vi "LinearPlntInvFF_New.vi"(5 "States":i32, 6 "dT_Seconds":dbl=0.02, 7 "Inputs":i32, 10 "B":T1, 11 "A":T1) -> (0 "Error":bool, 3 "Linear Plnt Inversion FF":T2)   [LabVIEW 2019, in "Trajectory_Library.lvlib"]
doc: "Creates a new LINEAR PLANT INVERSION FEEDFORWARD data cluster with the specified values. \n\n\nInputs: \n - XXX -- XXX.\n\nOutputs:\n - XXX -- XXX."
uses:
  Trajectory_Library.lvlib
  LINEAR_PLANT_INV_FF.ctl
  <vilib>/Analysis/Matrix/Datatypes/RealMatrix.ctl
  <vilib>/Analysis/Matrix/Numeric/Multiply/Multiply.vi
  <vilib>/Analysis/Matrix/Numeric/Multiply/Multiply - RM,R.vi
  Matrix_AssignBlock.vi
  Matrix_Exp.vi
  Matrix_ExtractFrom.vi
  <vilib>/Analysis/Matrix/NI_Matrix.lvlib
panel:
  # "<States,1>"
  # "<Inputs,1>"
  # "<States,Inputs>"
  # "<States,States>"
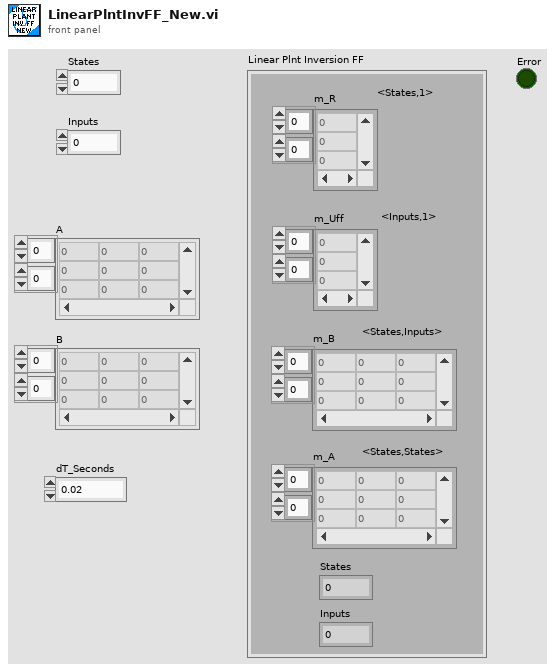
[diagram p1: front panel]
types:
  T1 = typedef "NI_Matrix.lvlib/RealMatrix.ctl" = dbl[][]
  T2 = typedef "Trajectory_Library.lvlib/LINEAR_PLANT_INV_FF.ctl" = cluster{"m_R":T1, "m_Uff":T1, "m_B":T1, "m_A":T1, "States":i32, "Inputs":i32}
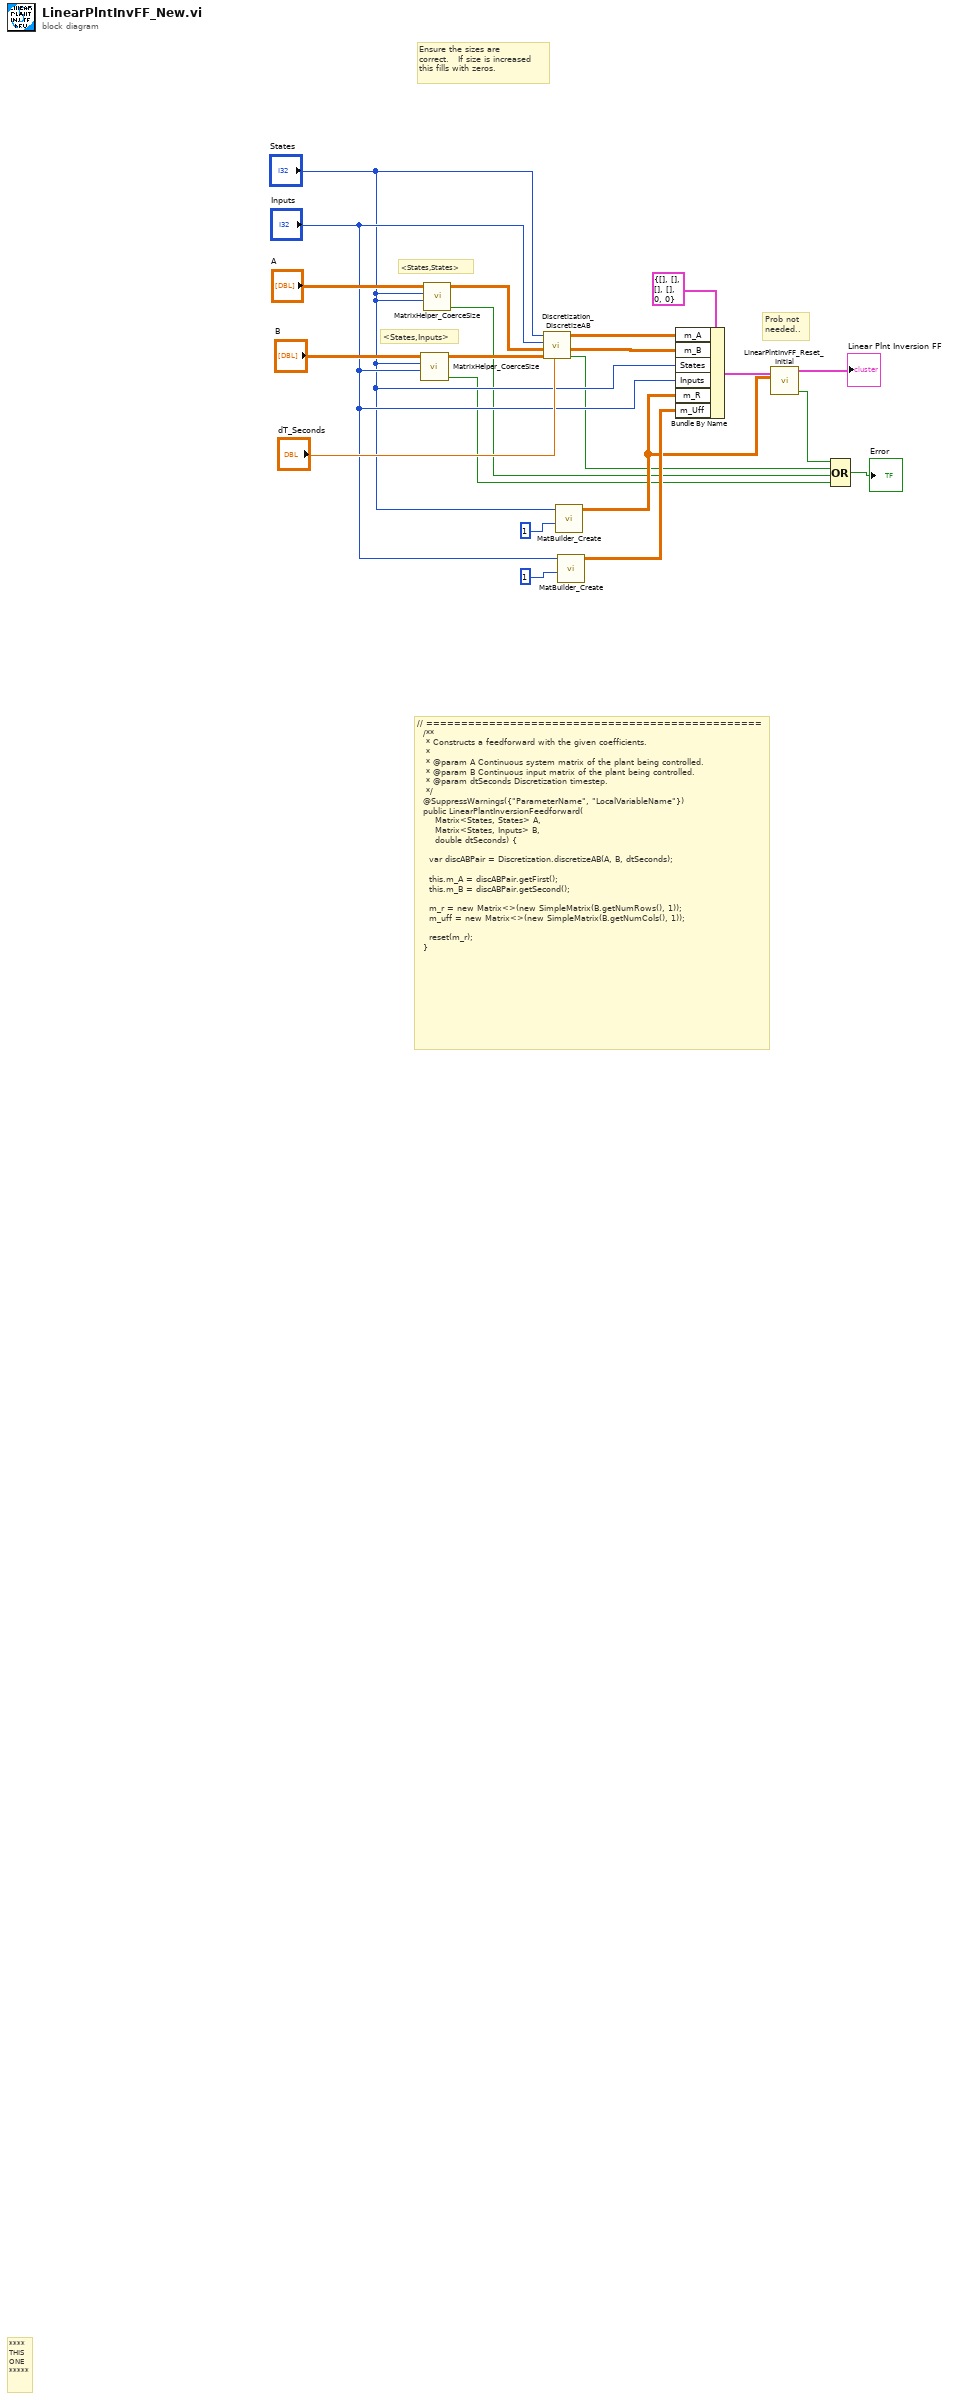
[diagram p0: block diagram]
diagram:
  # "Prob not \nneeded.."
  # "// ================================================\n  /**\n   * Constructs a feedforward with the given coefficients.\n   *\n   * @param A Continuous system matrix of the plant being controlled.\n   * @param B Continuous input matrix of the plant being controlled.\n   * @param dtSeconds Discretization timestep.\n   */\n  @SuppressWarnings({\"ParameterName\", \"LocalVariableName\"})\n  public LinearPlantInversionFeedforward(\n      Matrix<States, States> A, \n      Matrix<States, Inputs> B, \n      double dtSeconds) {\n\n    var discABPair = Discretization.discretizeAB(A, B, dtSeconds);\n \n    this.m_A = discABPair.getFirst();\n    this.m_B = discABPair.getSecond();\n\n    m_r = new Matrix<>(new SimpleMatrix(B.getNumRows(), 1));\n    m_uff = new Matrix<>(new SimpleMatrix(B.getNumCols(), 1));\n\n    reset(m_r);\n  }"
  # "<States,Inputs>"
  # "<States,States>"
  # "Ensure the sizes are\ncorrect.   If size is increased \nthis fills with zeros."
  # "****\nTHIS\nONE\n*****"
  n1 = call "MatrixHelper_CoerceSize.vi"("Columns"="Inputs", "Rows"="States", "input matrix"="B") -> ("Coerced"=w2:bool, "output matrix"=w12:T1)  [unwired: 7 in]
  n2 = call "MatrixHelper_CoerceSize.vi"("Columns"="States", "Rows"="States", "input matrix"="A") -> ("Coerced"=w3:bool, "output matrix"=w14:T1)  [unwired: 7 in]
  n3 = call "Discretization_DiscretizeAB.vi"("dT_Seconds"="dT_Seconds", "ContB"=w12, "ContA"=w14, "Inputs"="Inputs", "States"="States") -> ("Error"=w4:bool, "DiscB"=w18:T1, "DiscA"=w19:T1)  [unwired: 4 in]
  n4 = call "MatBuilder_Create.vi"("Columns"=1 ("number of columns"), "Rows"="States") -> ("output matrix"=w8:T1)  [unwired: 9 in]
  n5 = call "MatBuilder_Create.vi"("Columns"=1 ("number of columns"), "Rows"="Inputs") -> ("output matrix"=w11:T1)  [unwired: 9 in]
  n6 = Bundle By Name(cluster=T2 {"m_R"=[], "m_Uff"=[], "m_B"=[], "m_A"=[], "States"=0, "Inputs"=0} ("LINEAR_PLANT_INV_FF"), "m_A"=w19, "m_B"=w18, "States"="States", "Inputs"="Inputs", "m_R"=w8, "m_Uff"=w11) -> (w17:T2)
  n7 = call "LinearPlntInvFF_Reset_Initial.vi"("initialState"=w8, "Input Linear Plant Inv FF"=w17) -> ("Size Coerced"=w1:bool, "Output Linear Plant Inv FF"=→"Linear Plnt Inversion FF":T2)  [unwired: 8 in]
  n8 = Compound Arithmetic op=OR(w1, w4, w3, w2) -> (→"Error":bool)
